vi "Get XY Plot.vi"(8 "error in (no error)":errorcluster, 10 "Channel":u8, 11 "Instrument Driver in":refnum<class "Instrument Driver.lvclass">) -> (0 "error out":errorcluster, 2 "XY Plot":cluster{dbl[], "Spectrum, db":dbl[]}[](graph), 3 "Instrument Driver out":refnum<class "Instrument Driver.lvclass">)   [LabVIEW 2024, in "Instrument Driver.lvclass"]
uses:
  Instrument Driver.lvclass
  Instrument Driver.lvclass/Instrument Driver.ctl
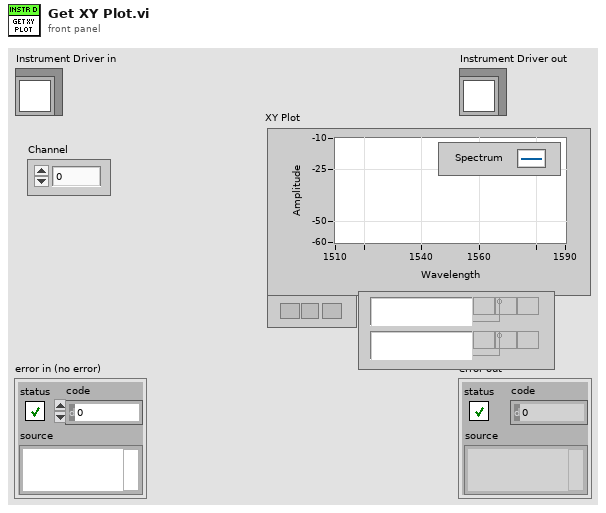
[diagram p1: front panel]
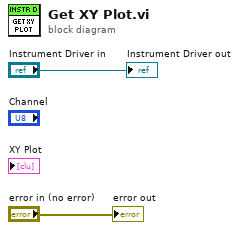
[diagram p0: block diagram]
diagram:
  "error out" <- "error in (no error)"
  "Instrument Driver out" <- "Instrument Driver in"
